vi "FFT_and_FindPeak_for_OneToneChannel_20190705.vi"(5 "Now.Target":T1=enum."4", 7 "DynRange_Thresh":dbl, 8 "CalTone?":bool, 10 "f":dbl, 11 "Tone In":T2={"Shift_"=0.0, "Peak_ToFPGA"=-24999462.633451957, "MaxValue"=0.0, "MaxIndex"=0, "Tone"={"PkLocTrak"=0.0, "PkLocDisp"=0.0, "df_"=0.0, "ZoomPwr"=[], "Phase"=0.0, "PhaseOld"=0.0, "AboveThresh?"=FALSE, "MaxI"=0.0, "MaxQ"=0.0, "median"=0.0, "ISpect"=[], "QSpect"=[], "DeltaPhase"=0.0}, "TimeDomainI"=[], "TimeDomainQ"=array[12500 elements], "PwrSpectrum"=[], "RunningAvgFreq"=0.0, "ISpectPos"=[], "ISpectNeg"=[], "QSpectPos"=[], "QSpectNeg"=[], "10Hz_PwrSpectr"=[], "SNR"=0.0, "AliasWarn"=FALSE, "10Hz_Peak"=[], "ISpect+-"=[], "QSpect+-"=[], "TimeStamp"=timestamp(0 s since 1904-01-01), "I_Index"=array[12500 elements], "Q_Index"=array[12500 elements], "10MHz"=FALSE} {"Tone"."median" format="%0.2f"; "Tone"."MaxQ" format="%0.2f"}) -> (0 "PeakLoc":dbl, 3 "Tone Out":T2={"Shift_"=0.0, "Peak_ToFPGA"=-24999462.633451957, "MaxValue"=0.0, "MaxIndex"=0, "Tone"={"PkLocTrak"=0.0, "PkLocDisp"=0.0, "df_"=0.0, "ZoomPwr"=[], "Phase"=0.0, "PhaseOld"=0.0, "AboveThresh?"=FALSE, "MaxI"=0.0, "MaxQ"=0.0, "median"=0.0, "ISpect"=[], "QSpect"=[], "DeltaPhase"=0.0}, "TimeDomainI"=[], "TimeDomainQ"=array[12500 elements], "PwrSpectrum"=[], "RunningAvgFreq"=0.0, "ISpectPos"=[], "ISpectNeg"=[], "QSpectPos"=[], "QSpectNeg"=[], "10Hz_PwrSpectr"=[], "SNR"=0.0, "AliasWarn"=FALSE, "10Hz_Peak"=[], "ISpect+-"=[], "QSpect+-"=[], "TimeStamp"=timestamp(0 s since 1904-01-01), "I_Index"=array[12500 elements], "Q_Index"=array[12500 elements], "10MHz"=FALSE} {"Tone"."median" format="%0.2f"; "Tone"."MaxQ" format="%0.2f"}, 4 "Shift_":dbl, 6 "x > y?":bool)   [LabVIEW 2018]
doc: "Perform FFT on ONE tone; either Cal or Beacon"
uses:
  Controls/ToneInfoClust.ctl
  Controls/Clusts/ChannelToneData.ctl
  Controls/Enums/TargetNumber.ctl
panel:
  out "RMS":dbl
  out "min value":dbl
  out "max value":dbl
  out "PeakValues":cluster{"IN":dbl, "IP":dbl, "QN":dbl, "QP":dbl}
  out "MaxIndex":i32
  out "Complex":dbl[](graph)
  out "Q":dbl[](graph)
  out "I":dbl[](graph)
  out "Power":dbl[](graph)
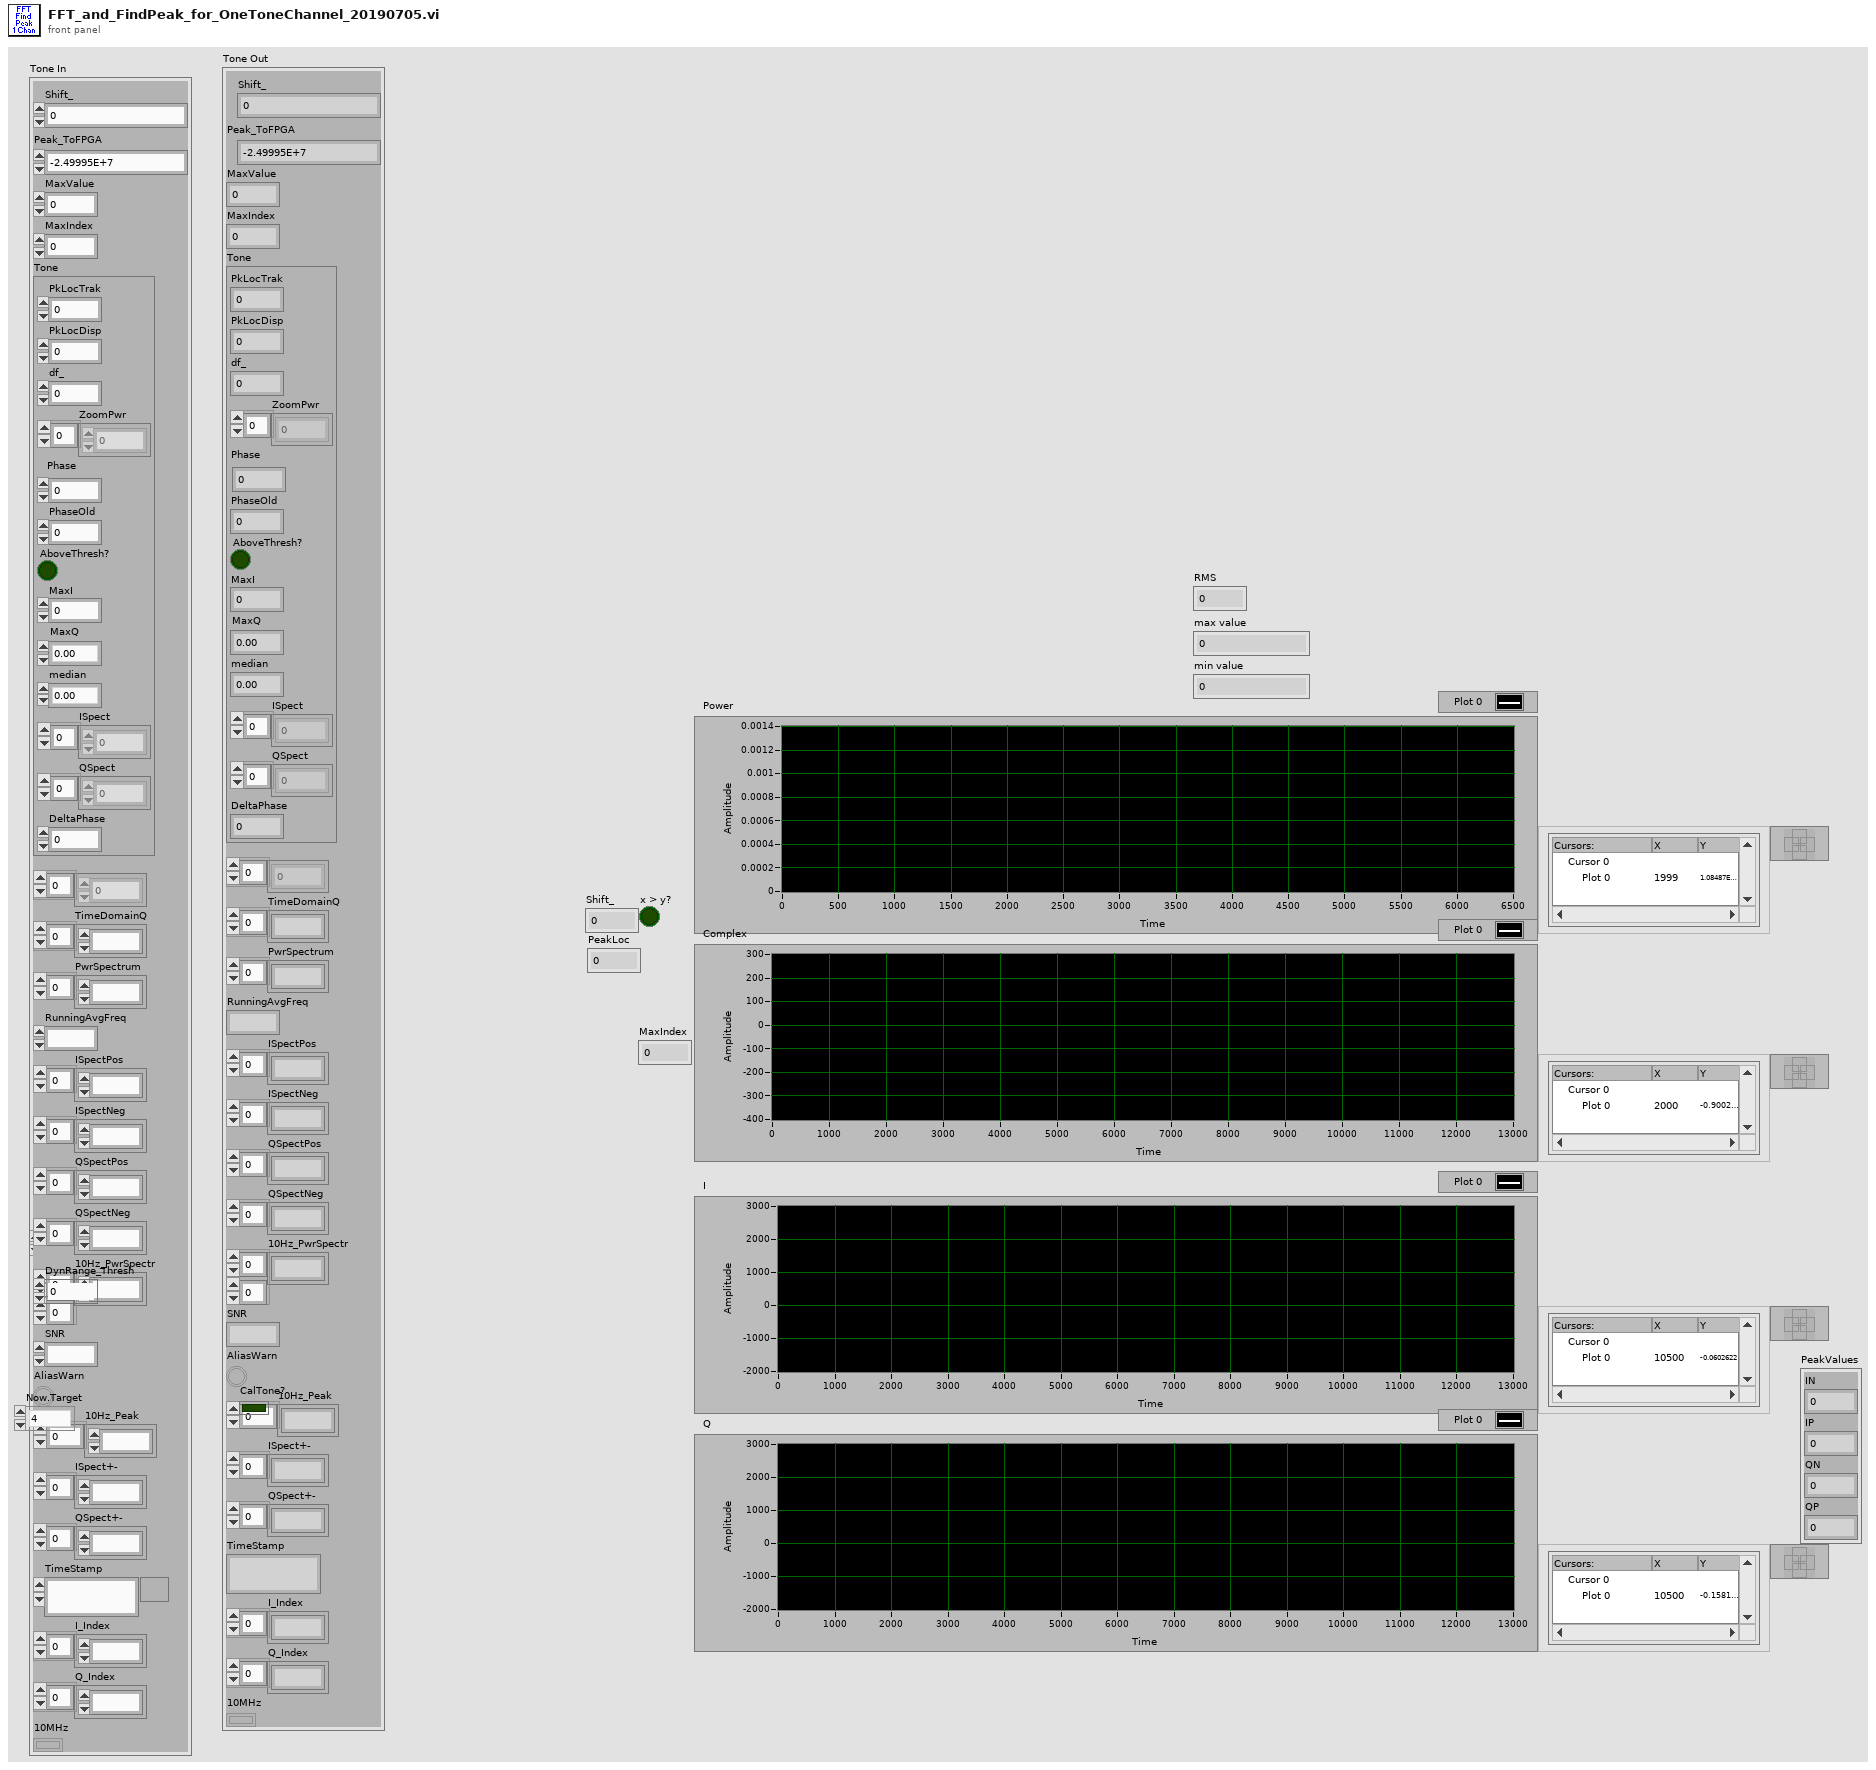
[diagram p1: front panel]
types:
  T1 = typedef "TargetNumber.ctl" = enum16{"1", "2", "3", "4"}
  T2 = typedef "ChannelToneData.ctl" = cluster{"Shift_":dbl, "Peak_ToFPGA":dbl, "MaxValue":dbl, "MaxIndex":i32, "Tone":T3, "TimeDomainI":ext[], "TimeDomainQ":ext[], "PwrSpectrum":dbl[], "RunningAvgFreq":dbl, "ISpectPos":dbl[], "ISpectNeg":dbl[], "QSpectPos":dbl[], "QSpectNeg":dbl[], "10Hz_PwrSpectr":dbl[][], "SNR":dbl, "AliasWarn":bool, "10Hz_Peak":dbl[], "ISpect+-":dbl[], "QSpect+-":dbl[], "TimeStamp":timestamp, "I_Index":ext[], "Q_Index":ext[], "10MHz":bool}
  T3 = typedef "ToneInfoClust.ctl" = cluster{"PkLocTrak":dbl, "PkLocDisp":dbl, "df_":dbl, "ZoomPwr":dbl[], "Phase":dbl, "PhaseOld":dbl, "AboveThresh?":bool, "MaxI":dbl, "MaxQ":dbl, "median":dbl, "ISpect":dbl[], "QSpect":dbl[], "DeltaPhase":dbl}
  T4 = typedef "ZoomSpectrumsClust.ctl" = cluster{"ZoomPowerSpectrum":dbl[], "MaxInPhase":dbl, "MaxQuadrature":dbl, "Phase":dbl, "ISpect":dbl[], "QSpect":dbl[]}
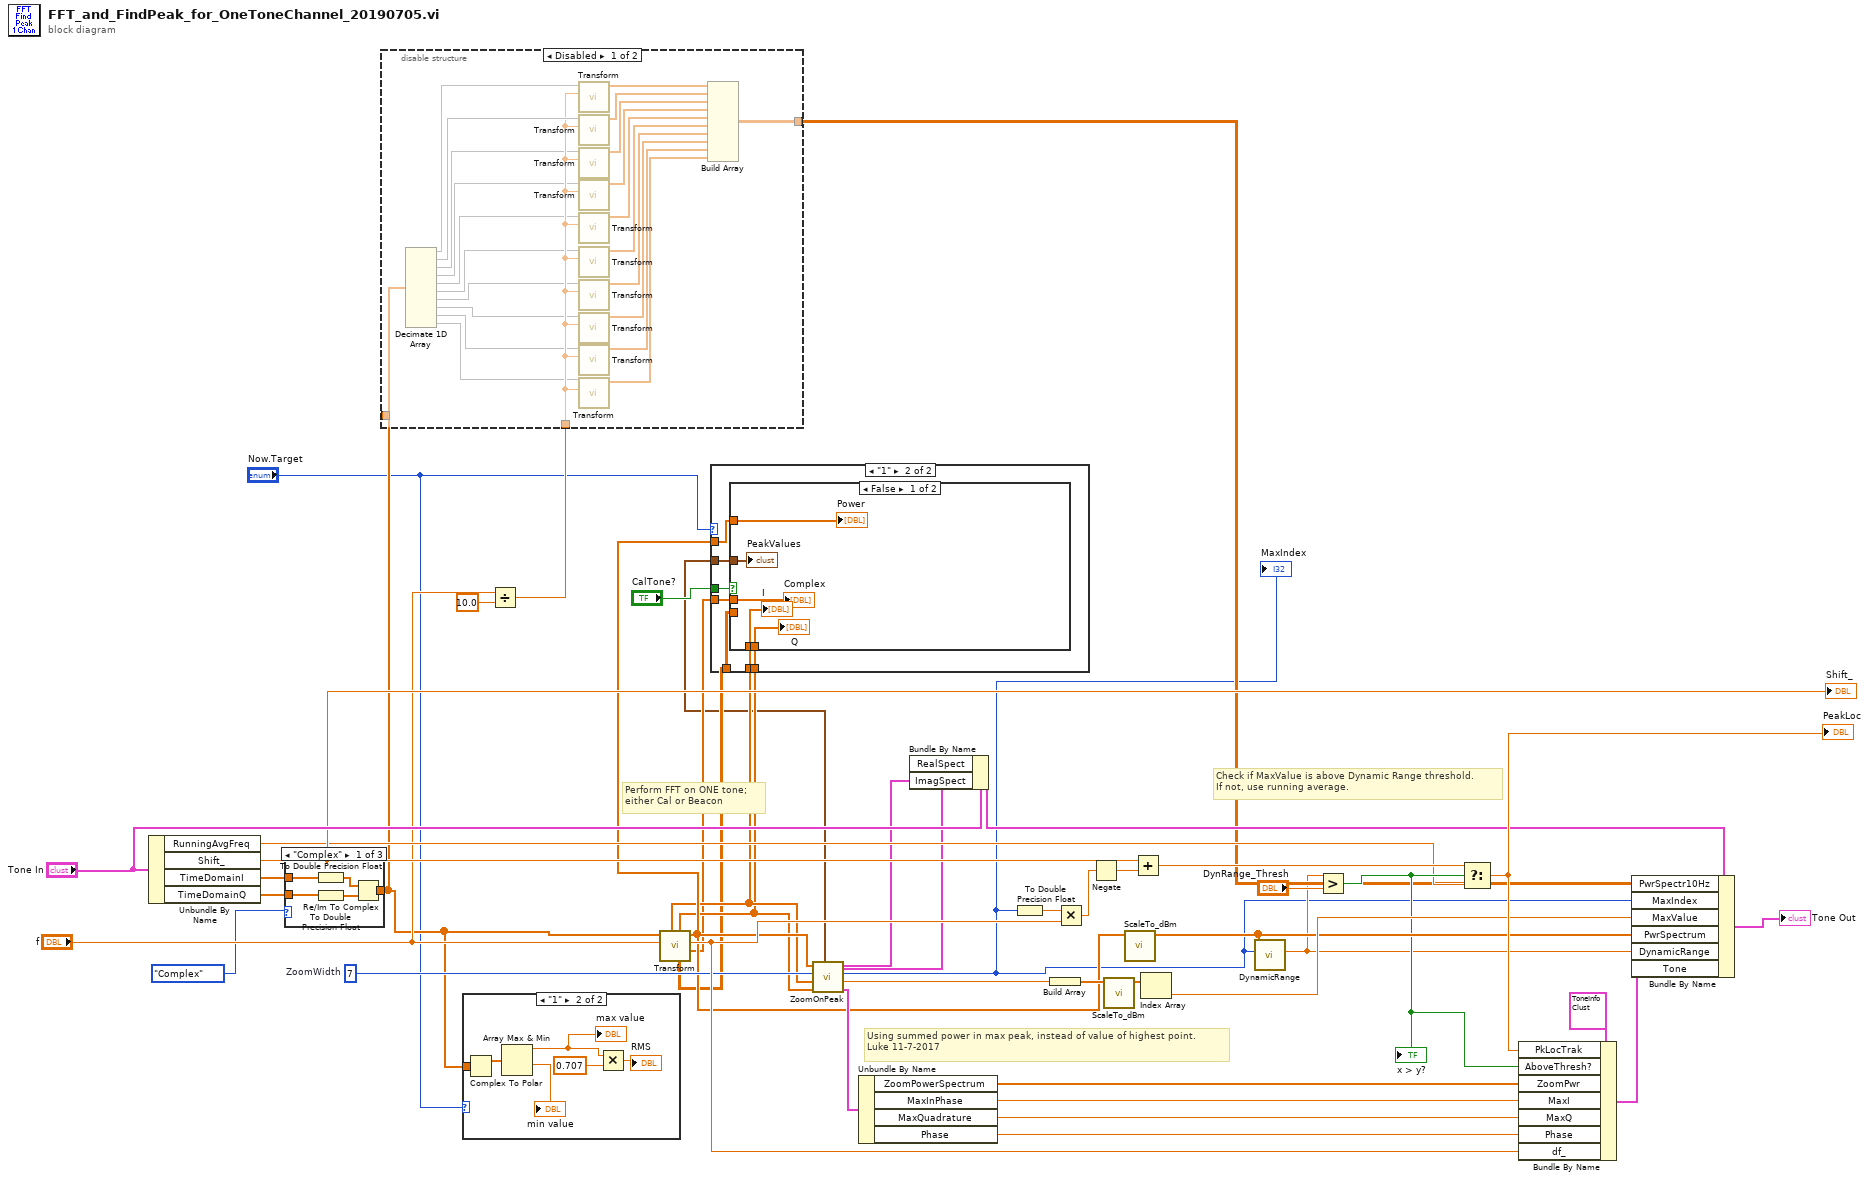
[diagram p0: block diagram]
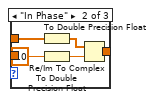
[diagram p4: hidden frame]
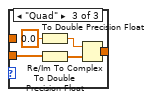
[diagram p5: hidden frame]
diagram:
  w41 = 7  # ZoomWidth
  # "Check if MaxValue is above Dynamic Range threshold.\nIf not, use running average."
  # "Using summed power in max peak, instead of value of highest point.\nLuke 11-7-2017"
  # "Perform FFT on ONE tone;\neither Cal or Beacon"
  n1 = Unbundle By Name("Tone In") -> ("RunningAvgFreq"=w28:dbl, "Shift_"=w30:dbl, "TimeDomainI"=w8:ext[], "TimeDomainQ"=w9:ext[])
  "Shift_" <- w30
  n2 = case shown="\"Complex\"" enum16{"Complex", "In Phase", "Quad"}."Complex" ("Enum") {
    tunnel: w9 -> [w49 _ w58]
    tunnel: [w48 w54 w59] -> w2
    tunnel: w8 -> [w47 w53 _]
    frame "Complex" {
      n3 = To Double Precision Float(number=w47) -> (double precision float=w51:dbl[])
      n4 = To Double Precision Float(number=w49) -> (double precision float=w50:dbl[])
      n5 = Re/Im To Complex(1:w50, 2:w51) -> (0:w48:cdb[])
    }
    frame "In Phase" {
      n6 = To Double Precision Float(number=w53) -> (double precision float=w56:dbl[])
      n7 = To Double Precision Float(number=0.0) -> (double precision float=w55:dbl)
      n8 = Re/Im To Complex(1:w55, 2:w56) -> (0:w54:cdb[])
    }
    frame "Quad" {
      n9 = To Double Precision Float(number=0.0) -> (double precision float=w61:dbl)
      n10 = To Double Precision Float(number=w58) -> (double precision float=w60:dbl[])
      n11 = Re/Im To Complex(1:w60, 2:w61) -> (0:w59:cdb[])
    }
  }
  n12 = case shown="\"1\"" "Now.Target" {
    tunnel: w2 -> [_ w67]
    frame Default {
    }
    frame "1" {
      n13 = Complex To Polar(r * e^(i*theta)=w67) -> (r=w66:dbl[])  [unwired: 1 out]
      n14 = Array Max & Min(array=w66) -> (max value=w64:dbl, min value=→"min value":dbl)  [unwired: 2 out]
      "max value" <- w64
      n15 = Multiply(x=w64, y=0.707) -> (x*y=→"RMS":dbl)
    }
  }
  n16 = Divide(x="f", y=10.0) -> (x/y=w13:dbl)
  n17 = disable-structure shown="Disabled" {
    disable-tunnel: w13 -> [w88 _]
    disable-tunnel: [w69 _] -> w12
    disable-tunnel: w2 -> [w68 _]
    frame Disabled {
      n18 = Decimate 1D Array(w68) -> (w90:cdb[], w89:cdb[], w87:cdb[], w86:cdb[], w85:cdb[], w84:cdb[], w83:cdb[], w82:cdb[], w81:cdb[], w80:cdb[])
      n19 = call "Transform.vi"("SampleRate"=w88, "TimeDomainIn"=w90) -> ("AmplitudeSpectrum"=w79:dbl[])  [unwired: 4 in, 5 out]
      n20 = call "Transform.vi"("SampleRate"=w88, "TimeDomainIn"=w89) -> ("AmplitudeSpectrum"=w78:dbl[])  [unwired: 4 in, 5 out]
      n21 = call "Transform.vi"("SampleRate"=w88, "TimeDomainIn"=w87) -> ("AmplitudeSpectrum"=w77:dbl[])  [unwired: 4 in, 5 out]
      n22 = call "Transform.vi"("SampleRate"=w88, "TimeDomainIn"=w86) -> ("AmplitudeSpectrum"=w76:dbl[])  [unwired: 4 in, 5 out]
      n23 = call "Transform.vi"("SampleRate"=w88, "TimeDomainIn"=w85) -> ("AmplitudeSpectrum"=w75:dbl[])  [unwired: 4 in, 5 out]
      n24 = call "Transform.vi"("SampleRate"=w88, "TimeDomainIn"=w84) -> ("AmplitudeSpectrum"=w74:dbl[])  [unwired: 4 in, 5 out]
      n25 = call "Transform.vi"("SampleRate"=w88, "TimeDomainIn"=w83) -> ("AmplitudeSpectrum"=w73:dbl[])  [unwired: 4 in, 5 out]
      n26 = call "Transform.vi"("SampleRate"=w88, "TimeDomainIn"=w82) -> ("AmplitudeSpectrum"=w72:dbl[])  [unwired: 4 in, 5 out]
      n27 = call "Transform.vi"("SampleRate"=w88, "TimeDomainIn"=w81) -> ("AmplitudeSpectrum"=w71:dbl[])  [unwired: 4 in, 5 out]
      n28 = call "Transform.vi"("SampleRate"=w88, "TimeDomainIn"=w80) -> ("AmplitudeSpectrum"=w70:dbl[])  [unwired: 4 in, 5 out]
      n29 = Build Array(w79, w78, w77, w76, w75, w74, w73, w72, w71, w70) -> (w69:dbl[][])
    }
    frame Enabled {
    }
  }
  n30 = call "Transform.vi"("SampleRate"="f", "TimeDomainIn"=w2) -> ("Complex"=w10:cdb[], "df (Hz)"=w46:dbl, "AmplitudeSpectrum"=w18:dbl[], "TheEugeneHong"=w6:dbl[][], "Quadrature"=w16:dbl[], "InPhase"=w17:dbl[])  [unwired: 4 in]
  n31 = call "ZoomOnPeak.vi"("Quadrature spectrum in"=w16, "InPhase spectrum in"=w17, "ZoomWidth"=w41, "Power spectrum in"=w18) -> ("ZoomSpectrs"=w24:T4, "Power of Peak"=w26:dbl, "MaxIndex"=w4:i32, "ZoomQ"=w25:cluster{"ZoomQPos":dbl[], "ZoomQNeg":dbl[]}, "ZoomI"=w27:cluster{"ZoomIPos":dbl[], "ZoomINeg":dbl[]}, "PeakValues"=w3:cluster{"IN":dbl, "IP":dbl, "QN":dbl, "QP":dbl})  [unwired: 2 in]
  "MaxIndex" <- w4
  n32 = case shown="\"1\"" "Now.Target" {
    tunnel: w18 -> [_ w97]
    tunnel: w17 -> [_ w96]
    tunnel: w16 -> [_ w95]
    tunnel: w10 -> [_ w94]
    tunnel: w6 -> [_ w93]
    tunnel: "CalTone?" -> [_ w92]
    tunnel: w3 -> [_ w91]
    frame Default {
    }
    frame "1" {
      n33 = case shown="False" w92 {
        tunnel: w97 -> [w102 _]
        tunnel: w96 -> [w101 _]
        tunnel: w95 -> [w100 _]
        tunnel: w94 -> [w99 _]
        tunnel: w93 -> [_ _]
        tunnel: w91 -> [w98 _]
        frame False {
          "Power" <- w102
          "I" <- w101
          "Q" <- w100
          "Complex" <- w99
          "PeakValues" <- w98
        }
        frame True {
        }
      }
    }
  }
  n34 = Unbundle By Name(w24) -> ("ZoomPowerSpectrum"=w23:dbl[], "MaxInPhase"=w22:dbl, "MaxQuadrature"=w21:dbl, "Phase"=w20:dbl)
  n35 = Bundle By Name(cluster="Tone In", "RealSpect"=w27, "ImagSpect"=w25) -> (w31:T2)
  n36 = To Double Precision Float(number=w4) -> (double precision float=w19:dbl)
  n37 = Build Array(w26) -> (w35:dbl[])
  n38 = Multiply(x=w19, y=w46) -> (x*y=w43:dbl)
  n39 = Negate(x=w43) -> (-x=w40:dbl)
  n40 = call "ScaleTo_dBm.vi"("PowerIn (unscaled)"=w35) -> ("PowerOut (dBm)"=w39:dbl[])  [unwired: 10 in]
  n41 = call "ScaleTo_dBm.vi"("PowerIn (unscaled)"=w18) -> ("PowerOut (dBm)"=w33:dbl[])  [unwired: 10 in]
  n42 = Add(x=w30, y=w40) -> (x+y=w37:dbl)
  n43 = Index Array(array=w39) -> (element=w34:dbl)  [unwired: 1 in]
  n44 = call "DynamicRange.vi"("MaxIndex"=w4, "Power (dBm)"=w33) -> ("DynamicRange"=w11:dbl)  [unwired: 8 in, 1 out]
  n45 = Greater?(x=w11, y="DynRange_Thresh") -> (0:w29:bool)
  "x > y?" <- w29
  n46 = Select(t=w37, s=w29, f=w28) -> (s? t:f=w36:dbl)
  "PeakLoc" <- w36
  n47 = Bundle By Name(cluster=T3 {"PkLocTrak"=0.0, "PkLocDisp"=0.0, "df_"=0.0, "ZoomPwr"=[], "Phase"=0.0, "PhaseOld"=0.0, "AboveThresh?"=FALSE, "MaxI"=0.0, "MaxQ"=0.0, "median"=0.0, "ISpect"=[], "QSpect"=[], "DeltaPhase"=0.0}, "PkLocTrak"=w36, "AboveThresh?"=w29, "ZoomPwr"=w23, "MaxI"=w22, "MaxQ"=w21, "Phase"=w20, "df_"=w46) -> (w44:T3)
  n48 = Bundle By Name(cluster=w31, "PwrSpectr10Hz"=w12, "MaxIndex"=w4, "MaxValue"=w34, "PwrSpectrum"=w33, "DynamicRange"=w11, "Tone"=w44) -> (→"Tone Out":T2)
